vi "APS initial.vi"(8 "error in (no error)":errorcluster caption="错误输入（无错误）", 10 "Mode":i32, 11 "BoardID_InBits":i32) -> (0 "error out":errorcluster caption="错误输出", 2 "function return":i32, 3 "BoardID_InBits out":i32)   [LabVIEW 2012, in "APS168.lvlib"]
doc: "I32 FNTYPE APS_initial( I32 *BoardID_InBits, I32 Mode );"
uses:
  APS168.lvlib
  APS168.dll
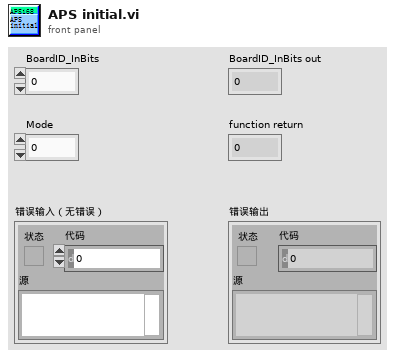
[diagram p1: front panel]
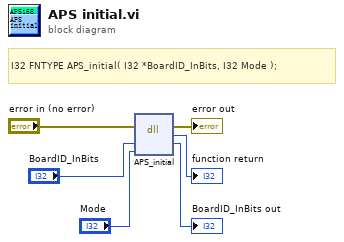
[diagram p0: block diagram]
diagram:
  # "I32 FNTYPE APS_initial( I32 *BoardID_InBits, I32 Mode );"
  n1 = dll-call lib="PTH1,abs E\t冲压机运动204c\nAPS168.dll" fn="APS_initial"(error in="error in (no error)", "BoardID_InBits"="BoardID_InBits", "Mode"="Mode") -> (error out=→"error out":errorcluster, "返回类型"=→"function return":i32, "BoardID_InBits"=→"BoardID_InBits out":i32)  [unwired: 3 in, 1 out]
